vi "KT2_SecondVI.vi"   [LabVIEW 2018]
uses:
  KT2/Paskevits_Vladislav_gbl1.vi
  KT2/Paskevits_Vladislav_gbl.vi
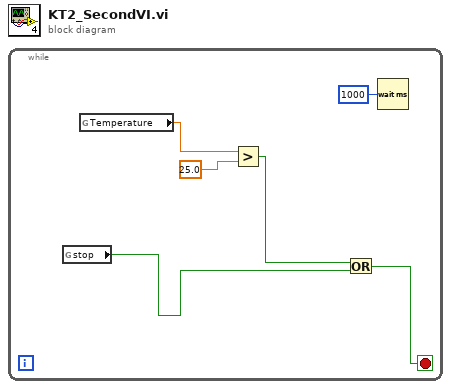
[diagram p0: block diagram]
diagram:
  n1 = while {
    stop <- w3 stop-if-true
    n2 = global read "Paskevits_Vladislav_gbl.vi" "stop"() -> (w1:bool)
    n3 = global read "Paskevits_Vladislav_gbl1.vi" "Temperature"() -> (w2:dbl)
    n4 = Greater?(x=w2, y=25.0) -> (0:w4:bool)
    n5 = Or(x=w4, y=w1) -> (x .or. y?=w3:bool)
    n6 = Wait (ms)(milliseconds to wait=u32 1000) -> ()  [unwired: 1 out]
  }
